vi "asset.attach_dataset_commit.vi"(8 "error in":errorcluster, 11 "AssetAttachDatasetStaging in":refnum<class "AssetAttachDatasetStaging.lvclass">) -> (0 "error out":errorcluster, 3 "AssetAttachDatasetStaging out":refnum<class "AssetAttachDatasetStaging.lvclass">)   [LabVIEW 2020, in "AssetAttachDatasetStaging.lvclass"]
doc: "Attaches the staged dataset, with its series-tag filters, to the asset and returns a handle to the updated asset."
uses:
  AssetAttachDatasetStaging.lvclass
  AssetAttachDatasetStaging.lvclass/AssetAttachDatasetStaging.ctl
  client.lvlib
panel:
  out "out_asset out":i32
  in  "rid":string
  in  "staging":i32
  in  "out_asset":i32
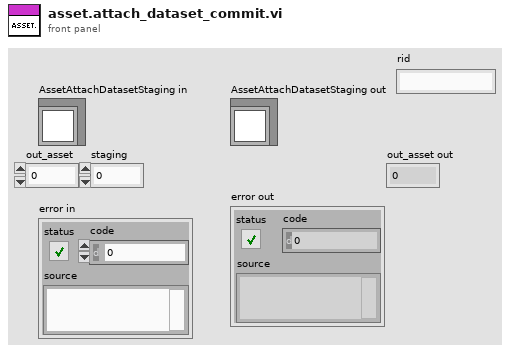
[diagram p1: front panel]
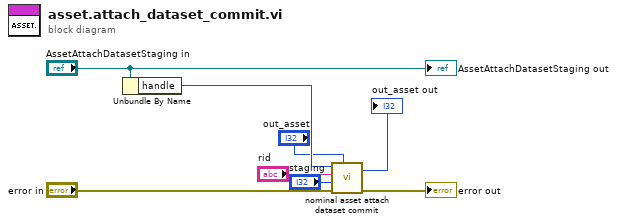
[diagram p0: block diagram]
diagram:
  n1 = Unbundle By Name("AssetAttachDatasetStaging in") -> ("handle"=w6:i32)
  n2 = call "nominal asset attach dataset commit.vi"("out_asset"="out_asset", "error in (no error)"="error in", "staging"="staging", "rid"="rid", "client"=w6) -> ("error out"=→"error out":errorcluster, "out_asset out"=→"out_asset out":i32)  [unwired: 4 in, 1 out]
  "AssetAttachDatasetStaging out" <- "AssetAttachDatasetStaging in"
